vi "SVT FFT Spectrum Subset (Mag-Phase) (1 Ch).vi"(0 "scaled signal [EU]":waveform(dbl)={"t0"=timestamp(0 s since 1904-01-01), "dt"=1e-05, "Y"=[]}, 2 "window":T8=1 items=["None"=0, "Hanning"=1, "Hamming"=2, "Blackman-Harris"=3, "Exact Blackman"=4, "Blackman"=5, "Flat Top"=6, "4 Term B-Harris "=7, "7 Term B-Harris"=8, "Low Sidelobe"=9, "Blackman Nuttall"=11, "Triangle"=30, "Bartlett-Hanning"=31, "Bohman"=32, "Parzen"=33, "Welch"=34, "Kaiser"=60, "Dolph-Chebyshev"=61, "Gaussian"=62], 3 "frequency range":T10={"start frequency"=1000.0, "stop frequency"=5000.0} {"stop frequency" min=0.0 format="%.2f"; "start frequency" min=0.0 format="%.2f"}, 4 "view":T1={"dB On (T)"=TRUE, "unwrap phase (F)"=FALSE, "convert to degree (T)"=TRUE}, 5 "error in (no error)":errorcluster, 7 "averaging parameters":T9={"averaging mode"=enum."No averaging", "weighting mode"=enum."Exponential", "number of averages"=10, "linear mode"=enum."One shot"}, 9 "restart averaging (F)":bool) -> (11 "averaging done":bool, 13 "averages completed":dbl=1.0, 14 "magnitude [dB EU]":cluster{"f0":dbl, "df":dbl, "magnitude":dbl[]}={"f0"=nan, "df"=inf, "magnitude"=[]} {"magnitude" format="%.2p"; "df" format="%.2p"; "f0" format="%.2p"}, 15 "magnitude unit label":string, 16 "phase [degrees]":cluster{"f0":dbl, "df":dbl, "phase":dbl[]}={"f0"=nan, "df"=inf, "phase"=[]} {"phase" format="%.2p"; "df" format="%.2p"; "f0" format="%.2p"}, 17 "phase unit label":string, 18 "spectrum info":T2={"channel name"="", "description"="", "x-axis units"=1, "spectral info"={"spectrum type"=enum."Power [Magnitude^2]", "linear/dB"=enum."linear", "window"=0, "window size"=0, "FFT size"=0}, "engineering units"=0, "custom label"="", "dB reference [EU]"=0.0, "peak units"=enum."rms", "weighting filter"=0, "spectral density?"=FALSE, "unit label"="", "spectrum skewed?"=FALSE, "complimentary spectrum units"=enum."none"} {"x-axis units" items=["Time (s)"=0, "Frequency-CB (Hz)"=1, "Frequency-CPB (Hz)"=1248, "Frequency-Arbitrary (Hz)"=2357, "Quefrency (s)"=2, "Revolutions (rev)"=3, "Order"=4, "Speed (RPM)"=11, "Speed (rad/s)"=21, "Index"=65535]; "weighting filter" items=["Linear", "A-weighting", "B-weighting", "C-weighting", "ITU-R 468-4", "Dolby", "CCITT", "C-message", "Wb", "Wc", "Wd", "We", "Wf", "Wh", "Wj", "Wk", "Wm", "AES17 20 kHz lowpass", "AES17 40 kHz lowpass", "AES17 20 kHz highpass", "AES17 40 kHz highpass"]; "dB reference [EU]" format="%.2f"; "engineering units" items=["custom..."=0, "V"=1, "A"=21, "C"=30, "pC"=31, "s"=32, "-"=29, "Pa"=2, "N"=20, "g"=3, "m/s^2"=4, "m/s"=5, "m"=6, "mm/s"=12, "mm"=13, "micron/s"=14, "micron"=15, "in/s^2"=7, "in/s"=8, "in"=9, "mil/s"=10, "mil"=11, "rad/s^2"=16, "rad/s"=17, "rad"=18, "deg/s^2"=26, "deg/s"=27, "deg"=28, "RPM"=22, "cycle/s^2"=23, "Hz"=24, "cycle"=25, "strain"=19]; "spectral info"."window" items=["None "=0, "Hanning"=1, "Hamming"=2, "Blackman-Harris"=3, "Exact Blackman"=4, "Blackman"=5, "Flat Top"=6, "4 Term B-Harris "=7, "7 Term B-Harris"=8, "Low Sidelobe"=9, "Force - Exponential"=10, "Gaussian"=62]}, 19 "error out":errorcluster)   [LabVIEW 2017]
doc: "Computes a subset of the FFT spectrum of <B>scaled signal [EU]</B>. The subset is defined by <B>frequency range</B>. FFT results are returned as <B>magnitude [dB EU]</B> and <B>phase [degrees]</B>. Each block of data corresponds to a single FFT block and has to be passed individually to this VI. You can use this polymorphic VI to analyze signals from a single channel or from N channels. The data type you wire to the <B>scaled signal [EU]</B> input determines the polymorphic instance to use."
uses:
  <vilib>/addons/_NISVFA/_Shared subVIs/Controls/svc_Window.ctl
  <vilib>/addons/_NISVFA/_Shared subVIs/Controls/svc_Spectrum Info.ctl
  <vilib>/addons/_NISVFA/_Shared subVIs/Controls/svc_X-Axis Units.ctl
  <vilib>/addons/_NISVFA/_Shared subVIs/Controls/svc_Spectrum Type.ctl
  <vilib>/addons/_NISVFA/_Shared subVIs/Controls/svc_Engineering Units Text Ring.ctl
  <vilib>/addons/_NISVFA/_Shared subVIs/Controls/svc_Weighting Filter Text Ring.ctl
  <vilib>/addons/_NISVFA/_Shared subVIs/Controls/svc_Complimentary Spectrum Units.ctl
  <vilib>/addons/_NISVFA/_Shared subVIs/Windowing/svfa_Scaled Time Domain Window (Array).vi
  <vilib>/addons/_NISVFA/_Shared subVIs/Common/svc_Get SV Channel Info.vi
  <vilib>/addons/_NISVFA/_Shared subVIs/Common/svc_Spectrum Units.vi
  <vilib>/addons/_NISVFA/_Shared subVIs/Spectrum Averaging/svfa_Reset Averaging State Info.vi
  <vilib>/addons/_NISVFA/_Shared subVIs/Spectrum Averaging/svfa_Average Array with Avg Checks (complex) No State.vi
  <vilib>/addons/_NISVFA/_Shared subVIs/Common/svc_Complex to Mag2 Array.vi
  <vilib>/addons/_NISVFA/_Shared subVIs/Spectrum Averaging/svfa_Average Array with Avg Checks (real) No State.vi
  <vilib>/Analysis/4window.llb/Force Window.vi
  <vilib>/Analysis/4window.llb/Force Window (DBL).vi
  <vilib>/Analysis/4window.llb/Exponential Window.vi
  <vilib>/Analysis/4window.llb/Exponential Window (DBL).vi
  <vilib>/addons/_NISVFA/_Shared subVIs/Spectrum Averaging/svfa_Average Array (complex) No State.vi
  <vilib>/addons/_NISVFA/_Shared subVIs/Spectrum Averaging/svfa_Average Array (real) No State.vi
  <vilib>/addons/_NISVFA/_Shared subVIs/Spectrum Averaging/svfa_No Average Array (complex).vi
  <vilib>/addons/_NISVFA/_Shared subVIs/Spectrum Averaging/svfa_Average Array (complex).vi
  <vilib>/addons/_NISVFA/_Shared subVIs/Spectrum Averaging/svfa_No Average Array (real).vi
  <vilib>/addons/_NISVFA/_Shared subVIs/Spectrum Averaging/svfa_Average Array (real).vi
  <vilib>/addons/_NISVFA/_Shared subVIs/Spectrum Averaging/svfa_Peak Hold Array.vi
  <vilib>/addons/_NISVFA/_Shared subVIs/Common/svc_Get Weighting Enum and Labels.vi
  <vilib>/addons/_NISVFA/_Shared subVIs/Common/svc_Unit Label Lexical Class.vi
  <vilib>/addons/_NISVFA/_Shared subVIs/Common/svc_Engineering Units to Unit Label.vi
  <vilib>/addons/_NISVFA/_Shared subVIs/Common/svc_Format Value (DBL).vi
  <vilib>/addons/_NISVFA/_Shared subVIs/Common/svc_Channel Info to Spectrum Info.vi
  <vilib>/addons/_NISVFA/_Shared subVIs/Common/svc_Unit Label to Engineering Units.vi
  <vilib>/Utility/error.llb/Error Cluster From Error Code.vi
  <vilib>/Analysis/0measdsp.llb/Scaled Time Domain Window.vi
  <vilib>/Analysis/0measdsp.llb/Scaled Time Domain Window (DBL).vi
  <vilib>/addons/_NISVFA/_Spectrum Processing/subVIs/svfa_Spectrum Info Window to windowTd Type Def.vi
  <vilib>/addons/_NISVFA/_Shared subVIs/Common/svc_Window Parameters.vi
  <vilib>/addons/_NISVFA/_Shared subVIs/Common/svc_Get Window Info.vi
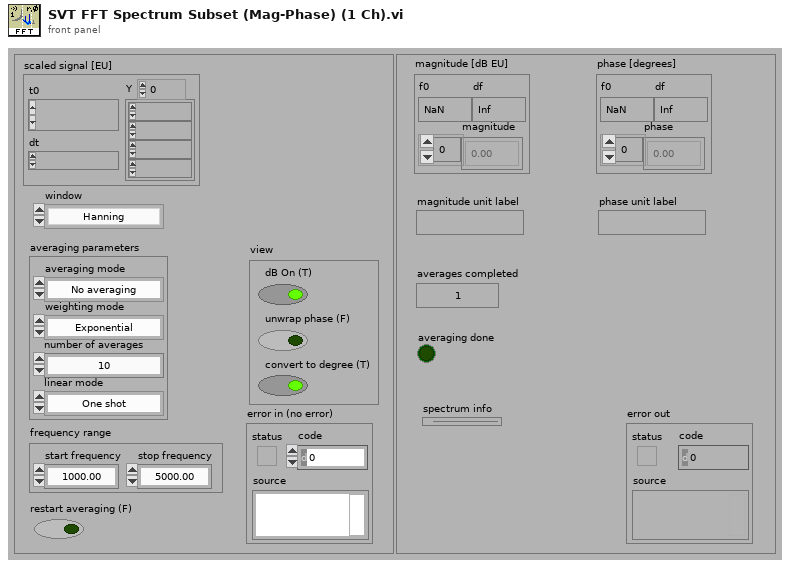
[diagram p1: front panel]
types:
  T1 = cluster{"dB On (T)":bool, "unwrap phase (F)":bool, "convert to degree (T)":bool}
  T2 = typedef "svc_Spectrum Info.ctl" = cluster{"channel name":string, "description":string, "x-axis units":T3, "spectral info":cluster{"spectrum type":T4, "linear/dB":enum16{"linear", "dB"}, "window":u16, "window size":i32, "FFT size":i32}, "engineering units":T5, "custom label":string, "dB reference [EU]":dbl, "peak units":enum16{"rms", "peak", "peak-peak"}, "weighting filter":T6, "spectral density?":bool, "unit label":string, "spectrum skewed?":bool, "complimentary spectrum units":T7}
  T3 = typedef "svc_X-Axis Units.ctl" = u16
  T4 = typedef "svc_Spectrum Type.ctl" = enum16{"FFT Spectrum [complex]", "Amplitude [Magnitude]", "Power [Magnitude^2]", "Cross Spectrum [complex]", "Frequency Response [Complex]"}
  T5 = typedef "svc_Engineering Units Text Ring.ctl" = u16
  T6 = typedef "svc_Weighting Filter Text Ring.ctl" = u16
  T7 = typedef "svc_Complimentary Spectrum Units.ctl" = enum16{"none", "radians", "degrees", "cycles", "imaginary"}
  T8 = typedef "svc_Window.ctl" = u32
  T9 = cluster{"averaging mode":enum16{"No averaging", "Vector averaging", "RMS averaging", "Peak hold"}, "weighting mode":enum16{"Linear", "Exponential"}, "number of averages":u32, "linear mode":enum16{"One shot", "Auto restart"}}
  T10 = cluster{"start frequency":dbl, "stop frequency":dbl}
  T11 = cluster{"f0":dbl, "df":dbl, "complex spectrum":cdb[]}
  T12 = enum16{"Restart processing", "Continue processing", "Skip processing"}
  T13 = enum16{"No averaging", "Vector averaging", "RMS averaging", "Peak hold"}
  T14 = cluster{"complex FFT":cdb[], "real FFT":dbl[], "f0":dbl, "df":dbl, "averages completed":dbl, "averaging parameters":cluster{"averaging mode":enum16{"No averaging", "Vector averaging", "RMS averaging", "Peak hold"}, "weighting mode":enum16{"Linear", "Exponential"}, "number of averages":u32, "linear mode":enum16{"One shot", "Auto restart"}}}
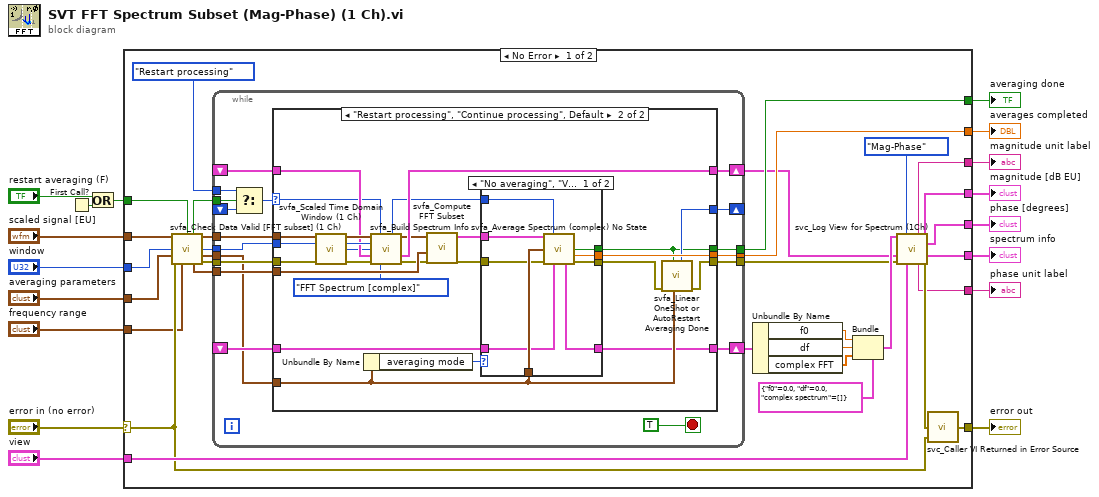
[diagram p0: block diagram]
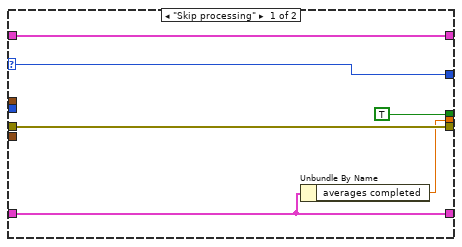
[diagram p2: hidden frame]
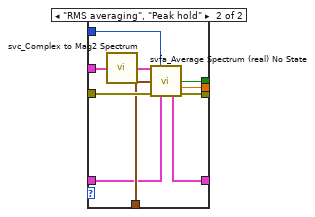
[diagram p3: hidden frame]
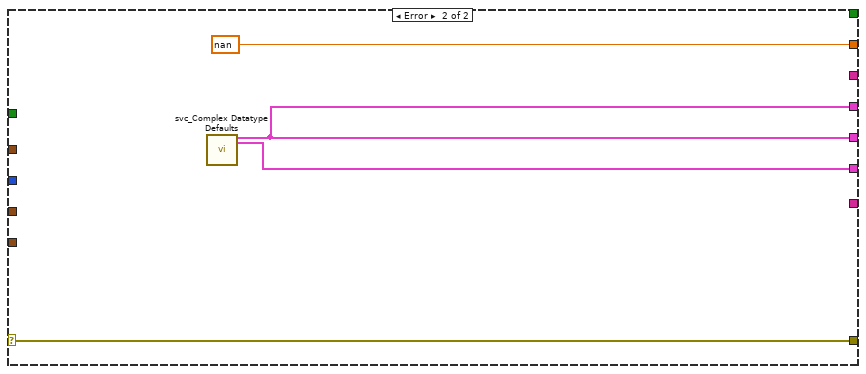
[diagram p4: hidden frame]
diagram:
  n1 = First Call?() -> (First Call?: T/F=w3:bool)
  n2 = Or(x="restart averaging (F)", y=w3) -> (x .or. y?=w2:bool)
  n3 = case shown="No Error" "error in (no error)" {
    selector: "error in (no error)" -> [w36 w122]
    tunnel: w2 -> [w48 _]
    tunnel: [w20 nan ("Averaged So-far")] -> w17
    tunnel: [w21 _] -> w16
    tunnel: [w38 w122] -> w15
    tunnel: "averaging parameters" -> [w45 _]
    tunnel: "frequency range" -> [w35 _]
    tunnel: "scaled signal [EU]" -> [w47 _]
    tunnel: "window" -> [w49 _]
    tunnel: [w42 w120] -> w4
    tunnel: [w41 _] -> w9
    tunnel: [w43 _] -> w8
    tunnel: "view" -> [w44 _]
    tunnel: [w40 w119] -> w6
    tunnel: [w39 w119] -> w5
    frame No Error {
      n4 = call <vilib>:"svfa_Check Data Valid [FFT subset] (1 Ch).vi"("signal"=w47, "restart averaging (F)"=w48, "window"=w49, "averaging parameters"=w45, "error in (no error)"=w36, "frequency range in"=w35) -> ("restart averaging"=w25:bool, "dup signal"=w30:waveform(dbl), "window"=w29:u16, "dup averaging parameters"=w26:T9, "frequency range out"=w28:T10, "error out"=w27:errorcluster)  [unwired: 4 in]
      n5 = while {
        shift-left: _ -> [w59]
        shift-right: [w60] -> w31
        tunnel: w28 -> [w62]
        tunnel: w30 -> [w63]
        tunnel: [w64] -> w20
        tunnel: [w66] -> w21
        tunnel: w27 -> [w67]
        tunnel: [w65] -> w22
        tunnel: w29 -> [w55]
        shift-right: [w57] -> w19
        shift-left: _ -> [w56]
        tunnel: w26 -> [w54]
        tunnel: w25 -> [w53]
        shift-right: [w61] -> _
        shift-left: _ -> [w52]
        tunnel: T12."Restart processing" ("processing control") -> [w51]
        stop <- TRUE stop-if-true
        n6 = Select(t=w51, s=w53, f=w52) -> (s? t:f=w50:T12)
        n7 = case shown="\"Restart processing\", \"Continue processing\", Default" w50 {
          selector: w50 -> [w71 w74]
          tunnel: w54 -> [_ w95]
          tunnel: [w70 w89] -> w60
          tunnel: w63 -> [_ w98]
          tunnel: w62 -> [_ w82]
          tunnel: [w71 w94] -> w61
          tunnel: w59 -> [w70 w88]
          tunnel: w55 -> [_ w96]
          tunnel: [w68 w79] -> w57
          tunnel: w56 -> [w68 w80]
          tunnel: [TRUE ("averaging done?") w91] -> w66
          tunnel: [w69 w99] -> w64
          tunnel: [w72 w93] -> w65
          tunnel: w67 -> [w72 w97]
          frame "Skip processing" {
            n8 = Unbundle By Name(w70) -> ("averages completed"=w69:dbl)
          }
          frame "Restart processing", "Continue processing", Default {
            n9 = call <vilib>:"svfa_Scaled Time Domain Window (1 Ch).vi"("Signal in [X]"=w98, "window"=w96, "error in"=w97) -> ("Windowed Waveform"=w85:waveform(dbl), "dup window"=w86:T8, "window length"=w76:i32, "error out"=w87:errorcluster)  [unwired: 7 in, 2 out]
            n10 = Unbundle By Name(w95) -> ("averaging mode"=w90:T13)
            n11 = call <vilib>:"svfa_Build Spectrum Info.vi"("scaled signal [EU]"=w85, "processing control"=w74, "window"=w86, "window size"=w76, "spectrum info in"=w80, "error in (no error)"=w87, "spectrum type"=svc_Spectrum_Type."FFT Spectrum [complex]" ("spectrum type 2")) -> ("dup processing control"=w78:T12, "dup scaled signal [EU]"=w75:waveform(dbl), "spectrum info out"=w79:T2, "error out"=w77:errorcluster)  [unwired: 5 in]
            n12 = call <vilib>:"svfa_Compute FFT Subset.vi"("error in (no error)"=w77, "frequency range"=w82, "windowed signal"=w75) -> ("error out"=w84:errorcluster, "FFT spectrum [Vrms]"=w83:cluster{"f0":dbl, "df":dbl, "spectrum":cdb[]})  [unwired: 7 in]
            n13 = case shown="\"No averaging\", \"Vector averaging\", Default" w90 {
              tunnel: w95 -> [w107 w115]
              tunnel: [w105 w111] -> w92
              tunnel: [w104 w117] -> w91
              tunnel: w83 -> [w108 w112]
              tunnel: w84 -> [w106 w118]
              tunnel: [w102 w116] -> w99
              tunnel: w78 -> [w103 w113]
              tunnel: [w101 w109] -> w89
              tunnel: w88 -> [w100 w110]
              frame "No averaging", "Vector averaging", Default {
                n14 = call <vilib>:"svfa_Average Spectrum (complex) No State.vi"("spectrum"=w108, "processing control"=w103, "averaging parameters"=w107, "error in (no error)"=w106, "averaging state info in"=w100) -> ("averaging done"=w104:bool, "averages completed"=w102:dbl, "averaging state info out"=w101:T14, "error out"=w105:errorcluster)  [unwired: 5 in, 2 out]
              }
              frame "RMS averaging", "Peak hold" {
                n15 = call <vilib>:"svc_Complex to Mag2 Spectrum.vi"("complex spectrum"=w112) -> ("power spectrum"=w114:cluster{"f0":dbl, "df":dbl, "spectrum":dbl[]})  [unwired: 4 in]
                n16 = call <vilib>:"svfa_Average Spectrum (real) No State.vi"("spectrum"=w114, "processing control"=w113, "averaging parameters"=w115, "error in (no error)"=w118, "averaging state info in"=w110) -> ("averaging done"=w117:bool, "averages completed"=w116:dbl, "averaging state info out"=w109:T14, "error out"=w111:errorcluster)  [unwired: 5 in, 2 out]
              }
            }
            n17 = call <vilib>:"svfa_Linear OneShot or AutoRestart Averaging Done.vi"("averaging parameters"=w95, "averaging done"=w91, "error in (no error)"=w92) -> ("error out"=w93:errorcluster, "processing control"=w94:T12)  [unwired: 7 in]
          }
        }
      }
      n18 = Unbundle By Name(w31) -> ("f0"=w34:dbl, "df"=w33:dbl, "complex FFT"=w32:cdb[])
      n19 = Bundle(cluster=T11 {"f0"=0.0, "df"=0.0, "complex spectrum"=[]} ("complex spectrum response"), "f0"=w34, "df"=w33, "complex spectrum"=w32) -> (w23:T11)
      n20 = call <vilib>:"svc_Log View for Spectrum (1Ch).vi"("complex spectrum"=w23, "View"=enum16{"Mag-Phase", "Real-Imaginary"}."Mag-Phase", "spectrum info in"=w19, "error in (no error)"=w22, "view"=w44) -> ("unit label [mag or real]"=w41:string, "magnitude or real"=w40:cluster{"f0":dbl, "df":dbl, dbl[]}, "phase or imag"=w39:cluster{"f0":dbl, "df":dbl, dbl[]}, "spectrum info out"=w42:T2, "unit label [phase or imag]"=w43:string, "error out"=w46:errorcluster)  [unwired: 5 in]
      n21 = call <vilib>:"svc_Caller VI Returned in Error Source.vi"("warning input to caller"=w36, "error in (no error)"=w46) -> ("error out"=w38:errorcluster)  [unwired: 3 in]
    }
    frame Error {
      n22 = call <vilib>:"svc_Complex Datatype Defaults.vi"() -> ("empty spectrum"=w119:cluster{"f0":dbl, "df":dbl, "magnitude":dbl[]}, "dead spectrum info"=w120:T2)  [unwired: 11 in, 7 out]
    }
  }
  "averages completed" <- w17
  "averaging done" <- w16
  "error out" <- w15
  "spectrum info" <- w4
  "magnitude unit label" <- w9
  "phase unit label" <- w8
  "magnitude [dB EU]" <- w6
  "phase [degrees]" <- w5
